vi "Entry.vi"(8 "error in (no error)":errorcluster, 11 "New State":refnum<class "Executing.lvclass">) -> (0 "error out":errorcluster, 3 "State out":refnum<class "Executing.lvclass">)   [LabVIEW 2013, in "Command Processor.lvlib" / "Executing.lvclass"]
doc: "This is an abstract method. Override this method to define the behavior when you enter the state."
uses:
  Executing.lvclass
  Command Processor.lvclass
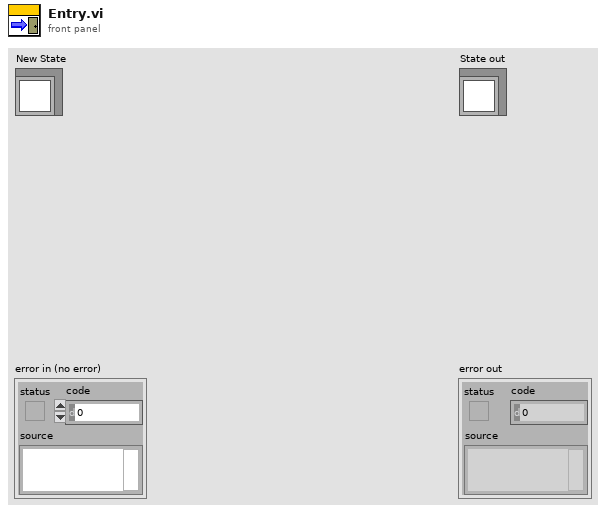
[diagram p1: front panel]
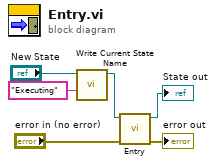
[diagram p0: block diagram]
diagram:
  n1 = call-dynamic "Write Current State Name.vi"("Current State Name"="Executing", "Command Processor in"="New State") -> ("Command Processor out"=w2:refnum<class "Executing.lvclass">)  [unwired: 8 in, 1 out]
  n2 = call-parent "Entry.vi"("error in (no error)"="error in (no error)", "New State"=w2) -> ("error out"=→"error out":errorcluster, "State out"=→"State out":refnum<class "Executing.lvclass">)  [unwired: 8 in]
